vi "Read Pages.vi"(8 "error in":errorcluster, 11 "Custom Device reference in":refnum<k24>) -> (0 "error out":errorcluster caption="error in", 2 "Pages":T1[](array[typedef]), 3 "Custom Device reference out":refnum<k24>)   [LabVIEW 2015, in "Configuration Tool.lvlib"]
uses:
  Configuration Tool.lvlib
  NationalInstruments.VeriStand.XMLReader
  XML Controls/Page.ctl
  XML Controls/Path Cluster.ctl
  XML Controls/Menu Item.ctl
  XML Controls/Execution Types.ctl
  XML Controls/Dependency three item small.ctl
  XML Controls/Button.ctl
  XML Controls/Button Type.ctl
  XML Controls/help.ctl
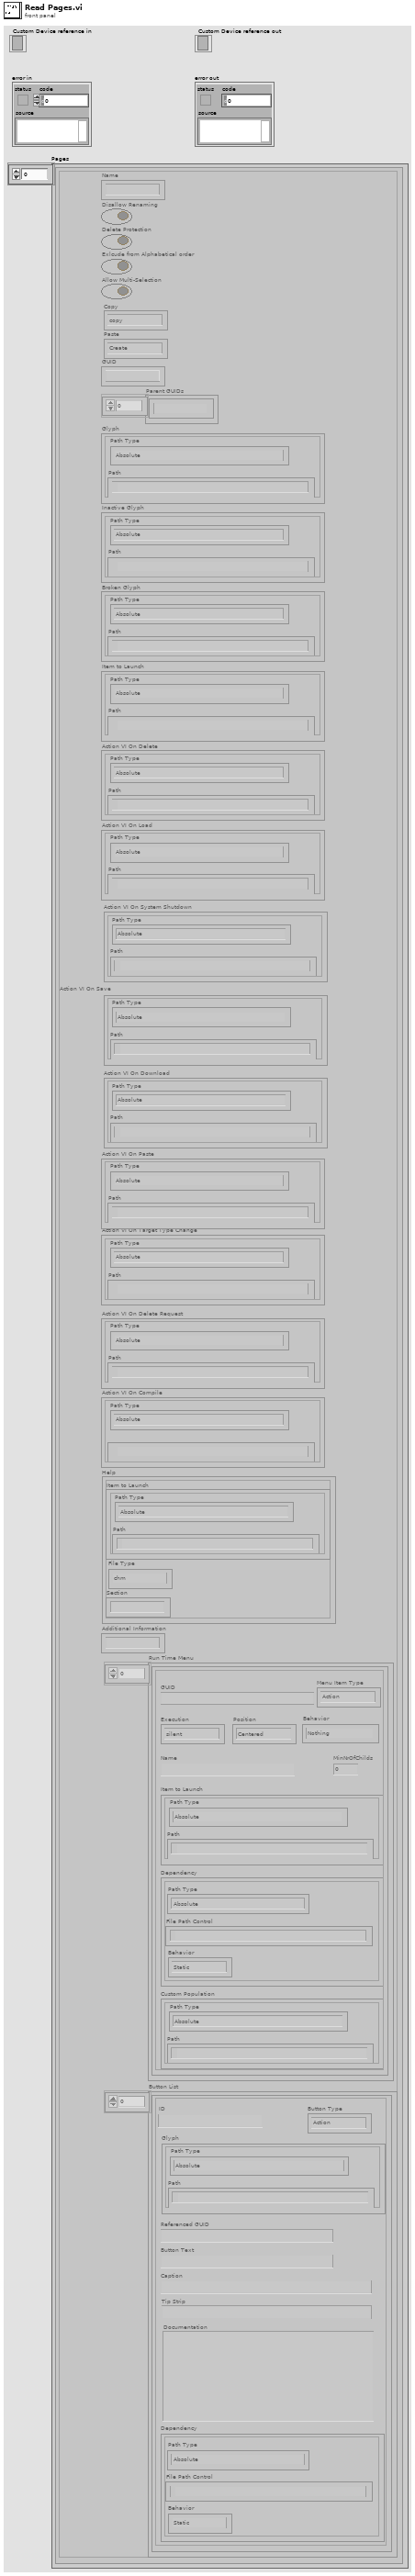
[diagram p1: front panel]
types:
  T1 = typedef "Configuration Tool.lvlib/Page.ctl" = cluster{"Name":string, "Disallow Renaming":bool, "Delete Protection":bool, "Exlcude from Alphabetical order":bool, "Allow Multi-Selection":bool, "GUID":string, "Parent GUIDs":string[], "Glyph":T2, "Inactive Glyph":T2, "Broken Glyph":T2, "Item to Launch":T2, "Action VI On Delete":T2, "Action VI On Load":T2, "Action VI On Paste":T2, "Action VI On Target Type Change":T2, "Action VI On Delete Request":T2, "Action VI On Compile":T2, "Additional Information":string, "Run Time Menu":T3[], "Button List":T6[], "Action VI On System Shutdown":T2, "Action VI On Save":T2, "Action VI On Download":T2, "Copy":enum16{"copy", "disabled"}, "Paste":enum16{"Create", "CreatIfNotExists_GUID", "CreatIfNotExists_Name", "Replace", "Dialog"}, "Help":T8}
  T2 = typedef "Configuration Tool.lvlib/Path Cluster.ctl" = cluster{"Path":path, "Path Type":enum16{"Absolute", "To Base", "To Common Doc Dir", "To Application Data Dir"}}
  T3 = typedef "Configuration Tool.lvlib/Menu Item.ctl" = cluster{"GUID":string, "Execution":T4, "MinNrOfChilds":u32, "Name":string, "Item to Launch":T2, "Dependency":T5, "Custom Population":T2, "Menu Item Type":enum16{"Action", "VI", "Separator", "Custom"}, "Behavior":enum16{"Nothing", "Open Front Panel"}, "Position":enum16{"Centered", "Mouse Pointer"}}
  T4 = typedef "Configuration Tool.lvlib/Execution Types.ctl" = enum16{"silent", "modal", "floating", "default"}
  T5 = typedef "Configuration Tool.lvlib/Dependency three item small.ctl" = cluster{"File Path Control":path, "Path Type":enum16{"Absolute", "To Base", "To Common Doc Dir", "To Application Data Dir"}, "Behavior":enum16{"Static", "Dynamic"}}
  T6 = typedef "Configuration Tool.lvlib/Button.ctl" = cluster{"ID":string, "Glyph":T2, "Button Type":T7, "Referenced GUID":string, "Button Text":string, "Caption":string, "Tip Strip":string, "Documentation":string, "Dependency":T5}
  T7 = typedef "Configuration Tool.lvlib/Button Type.ctl" = enum16{"Action", "Dialog", "Page", "Notification", "Separator"}
  T8 = typedef "Configuration Tool.lvlib/help.ctl" = cluster{"Item to Launch":T2, "Section":string, "File Type":enum16{"chm", "other"}}
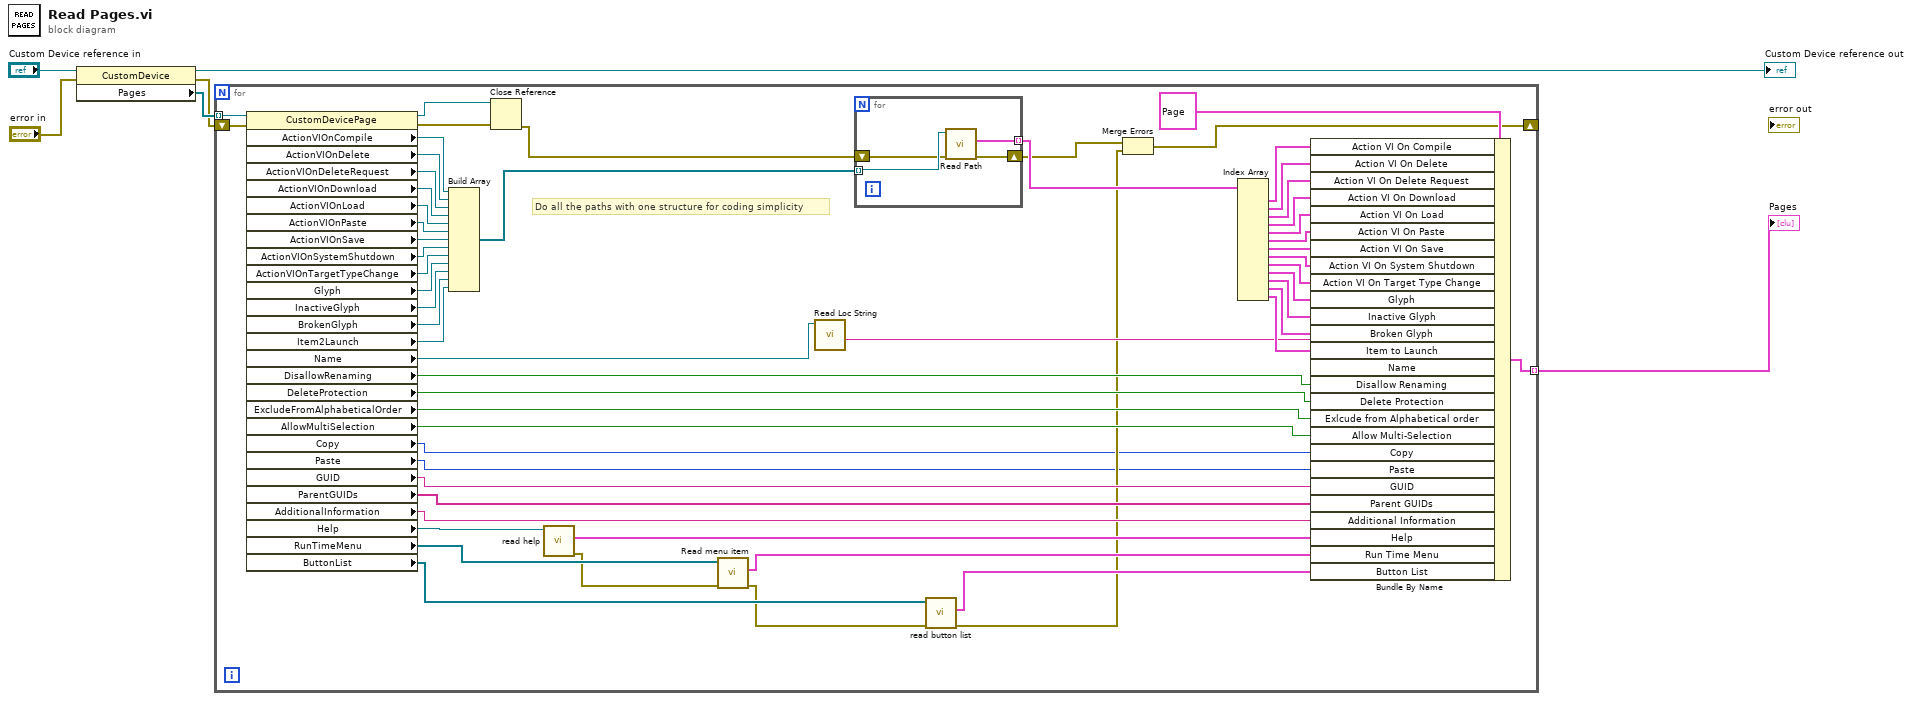
[diagram p0: block diagram]
diagram:
  n1 = property class="CustomDevice"(reference="Custom Device reference in", error in="error in") -> (reference out=→"Custom Device reference out":refnum<k24>, error out=w2:errorcluster, "Pages"=w4:refnum<k24>[])
  n2 = for {
    tunnel: w4 -> [w63] mode=indexing
    shift-right: [w9] -> _
    shift-left: w2 -> [w62]
    tunnel: [w51] -> w1 mode=indexing
    # "Do all the paths with one structure for coding simplicity"
    n3 = property class="CustomDevicePage"(reference=w63, error in=w62) -> (reference out=w49:refnum<k24>, error out=w48:errorcluster, "ActionVIOnCompile"=w60:refnum<k24>, "ActionVIOnDelete"=w59:refnum<k24>, "ActionVIOnDeleteRequest"=w58:refnum<k24>, "ActionVIOnDownload"=w57:refnum<k24>, "ActionVIOnLoad"=w56:refnum<k24>, "ActionVIOnPaste"=w55:refnum<k24>, "ActionVIOnSave"=w54:refnum<k24>, "ActionVIOnSystemShutdown"=w53:refnum<k24>, "ActionVIOnTargetTypeChange"=w52:refnum<k24>, "Glyph"=w32:refnum<k24>, "InactiveGlyph"=w31:refnum<k24>, "BrokenGlyph"=w30:refnum<k24>, "Item2Launch"=w29:refnum<k24>, "Name"=w28:refnum<k24>, "DisallowRenaming"=w26:bool, "DeleteProtection"=w25:bool, "ExcludeFromAlphabeticalOrder"=w24:bool, "AllowMultiSelection"=w23:bool, "Copy"=w8:i32, "Paste"=w7:i32, "GUID"=w22:string, "ParentGUIDs"=w21:string[], "AdditionalInformation"=w20:string, "Help"=w19:refnum<k24>, "RunTimeMenu"=w16:refnum<k24>[], "ButtonList"=w14:refnum<k24>[])
    n4 = Build Array(w60, w59, w58, w57, w56, w55, w54, w53, w52, w32, w31, w30, w29) -> (w50:refnum<k24>[])
    n5 = Close Reference(reference=w49, error in (no error)=w48) -> (error out=w47:errorcluster)
    n6 = call "read help.vi"(".NET Refnum in"=w19) -> ("error out"=w12:errorcluster, "Help"=w17:T8)  [unwired: 9 in]
    n7 = call "Read menu item.vi"("Error In"=w12, "RunTimeMenu"=w16) -> ("Error Out"=w11:errorcluster, "Run Time Menu"=w15:T3[])  [unwired: 8 in]
    n8 = call "Read Loc String.vi"(".NET Refnum in"=w28) -> ("loc"=w27:string)  [unwired: 8 in, 2 out]
    n9 = for {
      tunnel: w50 -> [w67] mode=indexing
      shift-right: [w65] -> w18
      shift-left: w47 -> [w66]
      tunnel: [w64] -> w46 mode=indexing
      n10 = call "Read Path.vi"("error in (no error)"=w66, "Path Ref"=w67) -> ("error out"=w65:errorcluster, "Path"=w64:T2)  [unwired: 8 in]
    }
    n11 = call "read button list.vi"("Error In"=w11, "ButtonList"=w14) -> ("Error Out"=w10:errorcluster, "Button List"=w13:T6[])  [unwired: 8 in]
    n12 = Merge Errors(w18, w10) -> (w9:errorcluster)
    n13 = Index Array(array=w46) -> (element #1=w45:T2, element #2=w44:T2, element #3=w43:T2, element #4=w42:T2, element #5=w41:T2, element #6=w40:T2, element #7=w39:T2, element #8=w38:T2, element #9=w37:T2, element #10=w36:T2, element #11=w35:T2, element #12=w34:T2, element #13=w33:T2)  [unwired: 13 in]
    n14 = Bundle By Name(cluster=T1 {"Name"="", "Disallow Renaming"=FALSE, "Delete Protection"=FALSE, "Exlcude from Alphabetical order"=FALSE, "Allow Multi-Selection"=FALSE, "GUID"="", "Parent GUIDs"=[], "Glyph"={"Path"=path "", "Path Type"=enum."Absolute"}, "Inactive Glyph"={"Path"=path "", "Path Type"=enum."Absolute"}, "Broken Glyph"={"Path"=path "", "Path Type"=enum."Absolute"}, "Item to Launch"={"Path"=path "", "Path Type"=enum."Absolute"}, "Action VI On Delete"={"Path"=path "", "Path Type"=enum."Absolute"}, "Action VI On Load"={"Path"=path "", "Path Type"=enum."Absolute"}, "Action VI On Paste"={"Path"=path "", "Path Type"=enum."Absolute"}, "Action VI On Target Type Change"={"Path"=path "", "Path Type"=enum."Absolute"}, "Action VI On Delete Request"={"Path"=path "", "Path Type"=enum."Absolute"}, "Action VI On Compile"={"Path"=path "", "Path Type"=enum."Absolute"}, "Additional Information"="", "Run Time Menu"=[], "Button List"=[], "Action VI On System Shutdown"={"Path"=path "", "Path Type"=enum."Absolute"}, "Action VI On Save"={"Path"=path "", "Path Type"=enum."Absolute"}, "Action VI On Download"={"Path"=path "", "Path Type"=enum."Absolute"}, "Copy"=enum."copy", "Paste"=enum."Create", "Help"={"Item to Launch"={"Path"=path "", "Path Type"=enum."Absolute"}, "Section"="", "File Type"=enum."chm"}} ("Page"), "Action VI On Compile"=w45, "Action VI On Delete"=w44, "Action VI On Delete Request"=w43, "Action VI On Download"=w42, "Action VI On Load"=w41, "Action VI On Paste"=w40, "Action VI On Save"=w39, "Action VI On System Shutdown"=w38, "Action VI On Target Type Change"=w37, "Glyph"=w36, "Inactive Glyph"=w35, "Broken Glyph"=w34, "Item to Launch"=w33, "Name"=w27, "Disallow Renaming"=w26, "Delete Protection"=w25, "Exlcude from Alphabetical order"=w24, "Allow Multi-Selection"=w23, "Copy"=w8, "Paste"=w7, "GUID"=w22, "Parent GUIDs"=w21, "Additional Information"=w20, "Help"=w17, "Run Time Menu"=w15, "Button List"=w13) -> (w51:T1)
  }
  "Pages" <- w1
